vi "Handle getAll.vi"(8 "error in (no error)":errorcluster, 11 "instrument.PPMS2 in":refnum<class "instrument.PPMS2.lvclass">) -> (0 "error out":errorcluster, 2 "getAll":variant, 3 "instrument.PPMS2 out":refnum<class "instrument.PPMS2.lvclass">)   [LabVIEW 2019, in "instrument.PPMS2.lvclass"]
uses:
  instrument.PPMS2.lvclass
  C:/Users/patrick/Documents/GitHub/PPMS-Monitor-and-Control/lvsrc/instrument.PPMS/instrument.PPMS.lvclass
  instrument.PPMS/Typedefs/PPMS.getAll--cluster.ctl
  instrument.PPMS/instrument.PPMS.lvclass
  C:/Program Files (x86)/National Instruments/LabVIEW 2019/user.lib/LevyLab/Instrument Framework/Instrument Types/Cryostat/Instrument.Cryostat.lvclass
  C:/Program Files (x86)/National Instruments/LabVIEW 2019/user.lib/LevyLab/Instrument Framework/SMOs/Instrument/Instrument.lvclass
  C:/Program Files (x86)/National Instruments/LabVIEW 2019/vi.lib/JKI/JKI SMO/SMO/SMO.lvclass
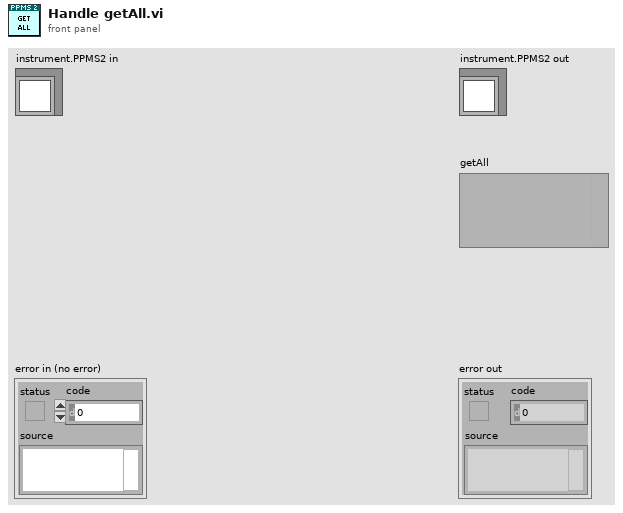
[diagram p1: front panel]
types:
  T1 = typedef "instrument.PPMS.lvclass/PPMS.getAll--cluster.ctl" = cluster{"Chamber Status":string, "Helium Level (%)":dbl, "Temperature (K)":dbl, "Temperature Status":string, "Magnetic Field (T)":dbl, "Magnet Status":string, "Position (°)":dbl}
  T2 = typedef "instrument.PPMS.lvclass/PPMS.Temperature Status--cluster.ctl" = cluster{"Temperature (K)":dbl, "Temperature Status":string}
  T3 = typedef "instrument.PPMS.lvclass/PPMS.Magnet Status--cluster.ctl" = cluster{"Field (T)":dbl, "Magnet Status":string}
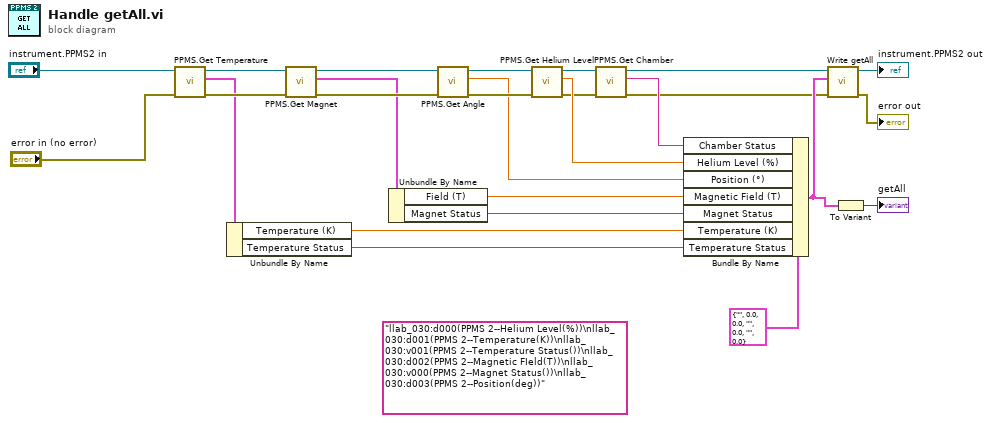
[diagram p0: block diagram]
diagram:
  (unwired) "llab_030:d000(PPMS 2--Helium Level(%))\nllab_030:d001(PPMS 2--Temperature(K))\nllab_030:v001(PPMS 2--Temperature Status())\nllab_030:d002(PPMS 2--Magnetic FIeld(T))\nllab_030:v000(PPMS 2--Magnet Status())\nllab_030:d003(PPMS 2--Position(deg))" ("Paths")
  n1 = call "PPMS.Get Temperature.vi"("error in (no error)"="error in (no error)", "instrument.PPMS"="instrument.PPMS2 in") -> ("error out"=w20:errorcluster, "Temperature Status"=w11:T2, "instrument.PPMS out"=w24:refnum<class "instrument.PPMS2.lvclass">)  [unwired: 7 in]
  n2 = Unbundle By Name(w11) -> ("Temperature (K)"=w13:dbl, "Temperature Status"=w12:string)
  n3 = call "PPMS.Get Magnet.vi"("error in (no error)"=w20, "instrument.PPMS"=w24) -> ("error out"=w19:errorcluster, "Magnet Status"=w16:T3, "instrument.PPMS out"=w23:refnum<class "instrument.PPMS2.lvclass">)  [unwired: 7 in]
  n4 = Unbundle By Name(w16) -> ("Field (T)"=w15:dbl, "Magnet Status"=w14:string)
  n5 = call "PPMS.Get Angle.vi"("error in (no error)"=w19, "instrument.PPMS"=w23) -> ("error out"=w18:errorcluster, "Angle (°)"=w17:dbl, "instrument.PPMS out"=w25:refnum<class "instrument.PPMS2.lvclass">)  [unwired: 7 in]
  n6 = call "PPMS.Get Helium Level.vi"("error in (no error)"=w18, "instrument.PPMS"=w25) -> ("error out"=w7:errorcluster, "Helium Level (%)"=w9:dbl, "instrument.PPMS out"=w8:refnum<class "instrument.PPMS2.lvclass">)  [unwired: 7 in]
  n7 = call "PPMS.Get Chamber.vi"("error in (no error)"=w7, "instrument.PPMS"=w8) -> ("error out"=w2:errorcluster, "Status String"=w6:string, "instrument.PPMS out"=w4:refnum<class "instrument.PPMS2.lvclass">)  [unwired: 7 in]
  n8 = Bundle By Name(cluster=T1 {"Chamber Status"="", "Helium Level (%)"=0.0, "Temperature (K)"=0.0, "Temperature Status"="", "Magnetic Field (T)"=0.0, "Magnet Status"="", "Position (°)"=0.0} ("getAll"), "Chamber Status"=w6, "Helium Level (%)"=w9, "Position (°)"=w17, "Magnetic Field (T)"=w15, "Magnet Status"=w14, "Temperature (K)"=w13, "Temperature Status"=w12) -> (w5:T1)
  n9 = call "Write getAll.vi"("error in (no error)"=w2, "getAll"=w5, "instrument.PPMS in"=w4) -> ("error out"=→"error out":errorcluster, "instrument.PPMS out"=→"instrument.PPMS2 out":refnum<class "instrument.PPMS2.lvclass">)  [unwired: 7 in]
  n10 = To Variant(anything=w5) -> (Variant=→"getAll":variant)
